vi "FGV.vi"(6 "Oper":T1(ring), 8 "error in":errorcluster, 9 "Waveforms":waveform(dbl)[](array[waveform]), 10 "Q-Name":string) -> (0 "error out":errorcluster, 1 "Waveforms":waveform(dbl)[](array[waveform]), 2 "All Datas":cluster{"Waveforms":waveform(dbl)[]}[](array[cluster]), 4 "Error":bool, 5 "Q-Names":string[](array[string]))   [LabVIEW 2016]
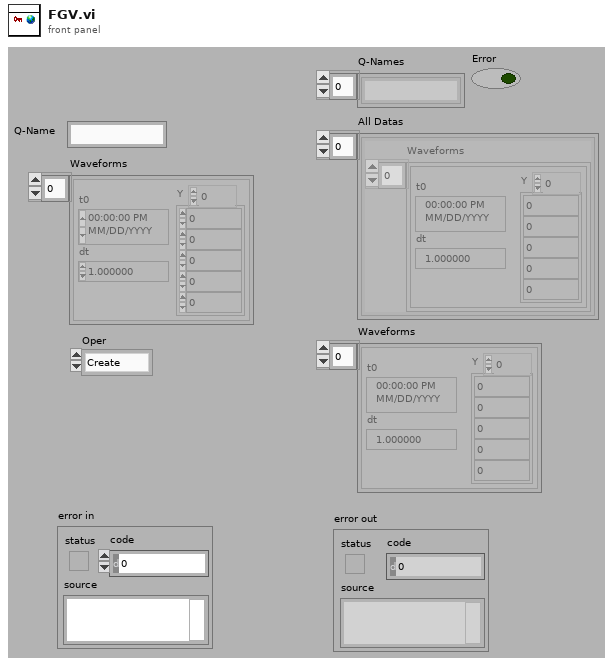
[diagram p1: front panel]
types:
  T1 = enum16{"Create", "Update", "New", "Get", "View", "Delete", "Close"}
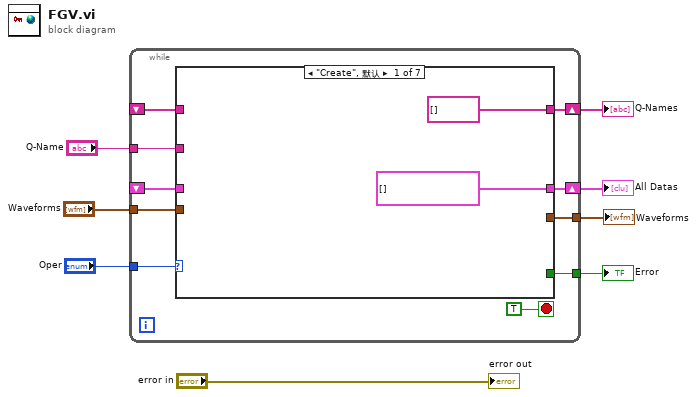
[diagram p0: block diagram]
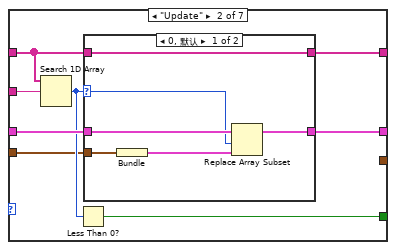
[diagram p2: hidden frame]
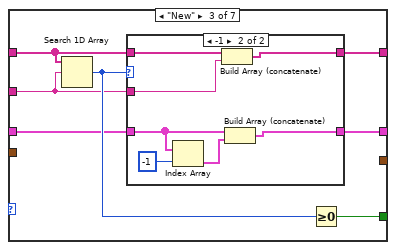
[diagram p4: hidden frame]
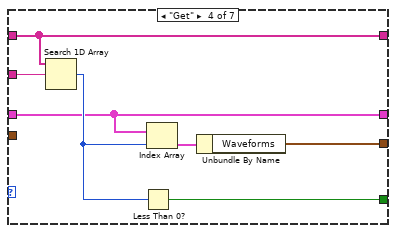
[diagram p6: hidden frame]
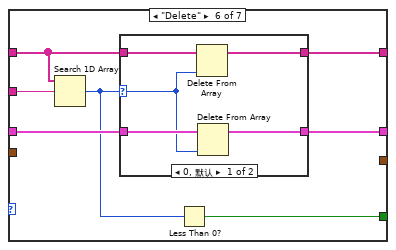
[diagram p8: hidden frame]
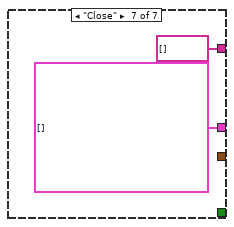
[diagram p10: hidden frame]
diagram:
  n1 = while {
    tunnel: "Oper" -> [w17]
    shift-right: [w16] -> w3
    shift-left: _ -> [w13]
    shift-right: [w15] -> w4
    shift-left: _ -> [w12]
    tunnel: "Q-Name" -> [w14]
    tunnel: "Waveforms" -> [w11]
    tunnel: [w10] -> w5
    tunnel: [w9] -> w2
    stop <- TRUE stop-if-true
    n2 = case shown="\"Create\", 默认" w17 {
      tunnel: [string[] [] w26 w39 w53 w60 w67 string[] []] -> w16
      tunnel: [cluster{"Waveforms":waveform(dbl)[]}[] [] ("All Datas") w24 w37 w54 w61 w65 cluster{"Waveforms":waveform(dbl)[]}[] [] ("All Datas")] -> w15
      tunnel: w14 -> [_ w28 w40 w59 _ w68 _]
      tunnel: w13 -> [_ w27 w42 w53 w60 w66 _]
      tunnel: w12 -> [_ w25 w38 w54 w61 w64 _]
      tunnel: w11 -> [_ w22 _ _ _ _ _]
      tunnel: [_ w21 w41 w58 _ w62 _] -> w10
      tunnel: [_ _ _ w55 _ _ _] -> w9
      frame "Create", Default {
      }
      frame "Update" {
        n3 = Search 1D Array(1D array=w27, element=w28) -> (index of element=w23:i32)  [unwired: 1 in]
        n4 = Less Than 0?(x=w23) -> (x < 0?=w21:bool)
        n5 = case shown="0, 默认" w23 {
          selector: w23 -> [w29 _]
          tunnel: w27 -> [w34 w36]
          tunnel: [w34 w36] -> w26
          tunnel: w25 -> [w33 w35]
          tunnel: [w32 w35] -> w24
          tunnel: w22 -> [w31 _]
          frame 0, Default {
            n6 = Bundle("Waveforms"=w31) -> (w30:cluster{"Waveforms":waveform(dbl)[]})  [unwired: 1 in]
            n7 = Replace Array Subset(array=w33, new element=w30, index=w29) -> (w32:cluster{"Waveforms":waveform(dbl)[]}[])
          }
          frame -1 {
          }
        }
      }
      frame "New" {
        n8 = Search 1D Array(1D array=w42, element=w40) -> (index of element=w43:i32)  [unwired: 1 in]
        n9 = case shown="-1" w43 {
          tunnel: w42 -> [w45 w52]
          tunnel: w40 -> [_ w51]
          tunnel: [w45 w50] -> w39
          tunnel: w38 -> [w44 w48]
          tunnel: [w44 w46] -> w37
          frame 0, Default {
          }
          frame -1 {
            n10 = Index Array(array=w48, index=-1) -> (element=w47:cluster{"Waveforms":waveform(dbl)[]})
            n11 = Build Array (concatenate)(w52, w51) -> (w50:string[])
            n12 = Build Array (concatenate)(w48, w47) -> (w46:cluster{"Waveforms":waveform(dbl)[]}[])
          }
        }
        n13 = Greater Or Equal To 0?(x=w43) -> (x >= 0?=w41:bool)
      }
      frame "Get" {
        n14 = Search 1D Array(1D array=w53, element=w59) -> (index of element=w57:i32)  [unwired: 1 in]
        n15 = Less Than 0?(x=w57) -> (x < 0?=w58:bool)
        n16 = Index Array(array=w54, index=w57) -> (element=w56:cluster{"Waveforms":waveform(dbl)[]})
        n17 = Unbundle By Name(w56) -> ("Waveforms"=w55:waveform(dbl)[])
      }
      frame "View" {
      }
      frame "Delete" {
        n18 = Search 1D Array(1D array=w66, element=w68) -> (index of element=w63:i32)  [unwired: 1 in]
        n19 = case shown="0, 默认" w63 {
          selector: w63 -> [w69 _]
          tunnel: [w72 w75] -> w67
          tunnel: w66 -> [w73 w75]
          tunnel: [w70 w74] -> w65
          tunnel: w64 -> [w71 w74]
          frame 0, Default {
            n20 = Delete From Array(array=w73, index=w69) -> (array with subset deleted=w72:string[])  [unwired: 1 in, 1 out]
            n21 = Delete From Array(array=w71, index=w69) -> (array with subset deleted=w70:cluster{"Waveforms":waveform(dbl)[]}[])  [unwired: 1 in, 1 out]
          }
          frame -1 {
          }
        }
        n22 = Less Than 0?(x=w63) -> (x < 0?=w62:bool)
      }
      frame "Close" {
      }
    }
  }
  "All Datas" <- w4
  "Waveforms" <- w2
  "Q-Names" <- w3
  "Error" <- w5
  "error out" <- "error in"
